vi "Aux3 Read 2016.vi"(7 "Array in":refnum<k24>[](array[refnum]), 8 "error in (no error)":errorcluster, 9 "Descriptions":string[](array[string]), 10 "Aux3 Slope In":dbl, 11 "Sensor Cluster":T1) -> (0 "error out":errorcluster, 2 "Sensor Cluster 2":T1, 3 "Aux3\\EC Out":dbl, 5 "Array out":refnum<k24>[](array[refnum]))   [LabVIEW 2016]
uses:
  controls/MCC DAQ Readings.ctl
  C:/Program Files/National Instruments/LabVIEW 2016/vi.lib/ULx/ULx_LV.dll
  Program Files/National Instruments/LabVIEW 2016/vi.lib/ULx/ULx_LV.dll
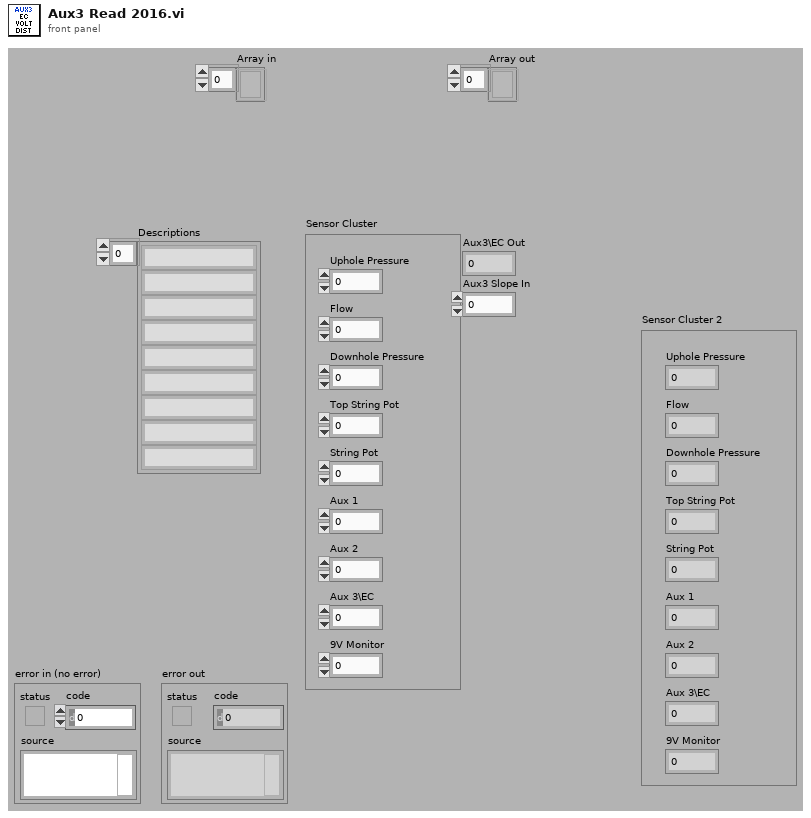
[diagram p1: front panel]
types:
  T1 = typedef "MCC DAQ Readings.ctl" = cluster{"Uphole Pressure":dbl, "Flow":dbl, "Downhole Pressure":dbl, "Top String Pot":dbl, "String Pot":dbl, "Aux 1":dbl, "Aux 2":dbl, "Aux 3\\EC":dbl, "9V Monitor":dbl}
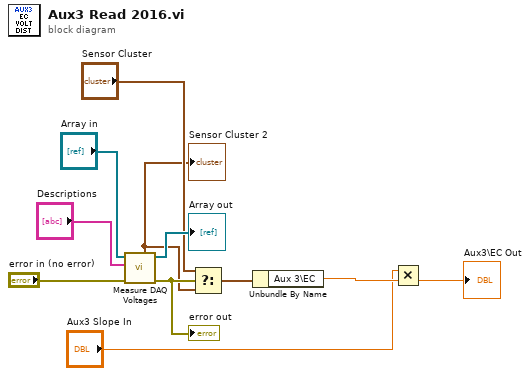
[diagram p0: block diagram]
diagram:
  n1 = call "Measure DAQ Voltages.vi"("error in (no error)"="error in (no error)", "Descriptions"="Descriptions", "Array in"="Array in") -> ("error in (no error) 2"=w6:errorcluster, "Array out"=→"Array out":refnum<k24>[], "Sensor Cluster"=w4:T1)  [unwired: 5 in, 1 out]
  "Sensor Cluster 2" <- w4
  "error out" <- w6
  n2 = Select(t="Sensor Cluster", s=w6, f=w4) -> (s? t:f=w3:T1)
  n3 = Unbundle By Name(w3) -> ("Aux 3\\EC"=w7:dbl)
  n4 = Multiply(x="Aux3 Slope In", y=w7) -> (x*y=→"Aux3\\EC Out":dbl)
